vi "levelStyleColorConfigurator.vi"(8 "error in (no error)":errorcluster, 11 "Colors in":u32[](array[numeric])) -> (0 "error out":errorcluster, 3 "Colors out":u32[](array[numeric]))   [LabVIEW 2017, in "Error Log.lvlib" / "Handler.UserEvent.Console.lvclass"]
uses:
  Handler.UserEvent.Console.lvclass
panel:
  in  "Cancel":bool
  in  "OK":bool
  in  "Colors":u32[](array[colorbox])
  out "Levels":T1(array[ring])=[enum."DEBUG", enum."INFO", enum."WARNING", enum."ERROR", enum."CRITICAL"]
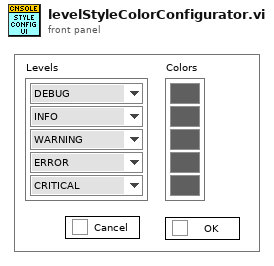
[diagram p1: front panel]
types:
  T1 = enum16{"DEBUG", "INFO", "WARNING", "ERROR", "CRITICAL"}[]
  T2 = enum32{"Invalid", "Standard", "Closed", "Hidden", "Minimized", "Maximized"}
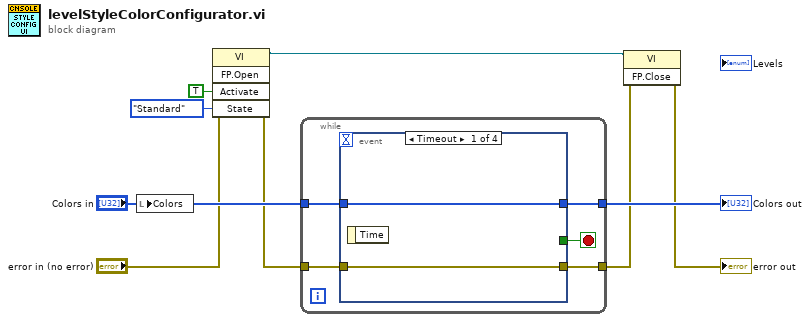
[diagram p0: block diagram]
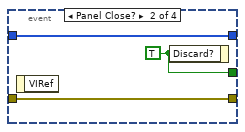
[diagram p2: hidden frame]
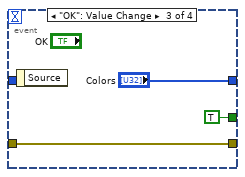
[diagram p3: hidden frame]
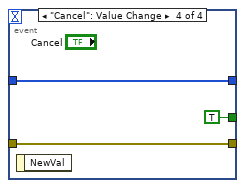
[diagram p4: hidden frame]
diagram:
  n1 = local write "Colors"("Colors in") -> ()
  n2 = invoke class="VI" method="FP.Open"(error in="error in (no error)", "Activate"=TRUE ("Activate?"), "State"=T2."Standard") -> (reference out=w5:refnum<vi>, error out=w6:errorcluster)  [unwired: 2 in, 3 out]
  n3 = while {
    tunnel: "Colors in" -> [w13]
    tunnel: w6 -> [w12]
    tunnel: [w11] -> w2
    tunnel: [w10] -> w9
    stop <- w14 stop-if-true
    n4 = event shown="[0] Timeout" {
      selector: _ -> [_ _ _ _]
      dyn-events: _ -> [_ _ _ _]
      timeout: _ -> [_ _ _ _]
      tunnel: [_ w19 TRUE ("Discard?") TRUE ("Discard?")] -> w14
      tunnel: w13 -> [w15 w17 _ w23]
      tunnel: w12 -> [w16 w18 w21 w24]
      tunnel: [w16 w18 w21 w24] -> w11
      tunnel: [w15 w17 "Colors" w23] -> w10
      event Timeout {
        n5 = event-data() -> ()  [unwired: 1 in, 1 out]
      }
      event Panel Close? {
        w19 = TRUE ("Discard?")
        n6 = event-data() -> ()  [unwired: 1 in, 1 out]
        n7 = event-data("Discard?"=w19) -> ()  [unwired: 1 in, 1 out]
      }
      event "OK": Value Change {
        n8 = event-data() -> ()  [unwired: 1 in, 1 out]
      }
      event "Cancel": Value Change {
        n9 = event-data() -> ()  [unwired: 1 in, 1 out]
      }
    }
  }
  "Colors out" <- w9
  n10 = invoke class="VI" method="FP.Close"(reference=w5, error in=w2) -> (error out=→"error out":errorcluster)  [unwired: 1 in, 2 out]
